vi "Set Exposure Manual.vi"(8 "error in":errorcluster, 11 "DMK33UP2000 in":refnum<class "DMK33UP2000.lvclass">) -> (0 "error out":errorcluster, 2 "Supported?":bool, 3 "DMK33UP2000 out":refnum<class "DMK33UP2000.lvclass">)   [LabVIEW 2018, in "DMK33UP2000.lvlib" / "DMK33UP2000.lvclass"]
uses:
  DMK33UP2000.lvclass
  builds/Camera.lvlibp/Camera.lvclass
  <resource>/objmgr/imaqdx.rc
  C:/Users/Ron.Dexter.LUMINARTECH/Desktop/builds/Camera.lvlibp/Camera.lvclass
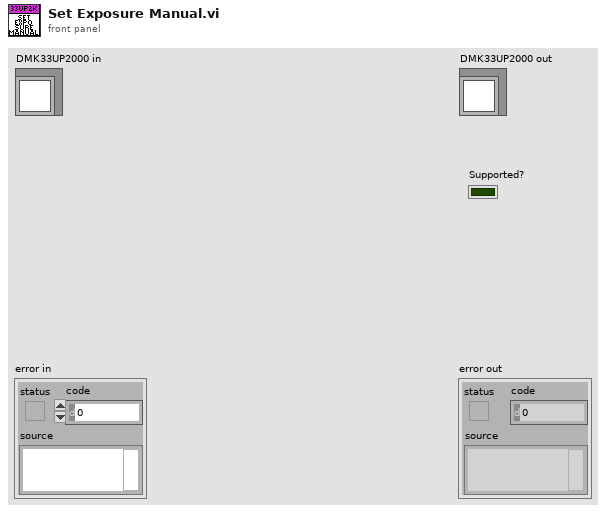
[diagram p1: front panel]
types:
  T1 = typedef "Camera.lvlibp/IMAQdx.ctl" = refnum<k21>
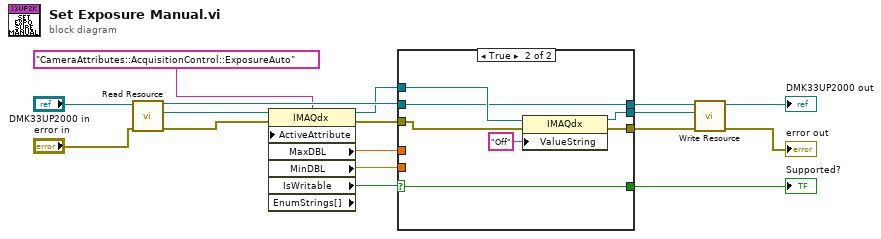
[diagram p0: block diagram]
diagram:
  n1 = call "Read Resource.vi"("error in (no error)"="error in", "Camera in"="DMK33UP2000 in") -> ("error out"=w8:errorcluster, "IMAQdx Session"=w7:T1, "Camera out"=w12:refnum<class "DMK33UP2000.lvclass">)  [unwired: 7 in]
  n2 = property class="IMAQdx" props=["ActiveAttribute", "MaxDBL", "MinDBL", "IsWritable", "EnumStrings[]"](reference=w7, error in=w8, "ActiveAttribute"="CameraAttributes::AcquisitionControl::ExposureAuto") -> (reference out=w10:T1, error out=w14:errorcluster, "MaxDBL"=w16:dbl, "MinDBL"=w17:dbl, "IsWritable"=w9:bool)  [unwired: 1 out]
  n3 = case shown="True" w9 {
    selector: w9 -> [w19 w28]
    tunnel: [w19 w28] -> w1
    tunnel: w10 -> [w20 w27]
    tunnel: [w20 w26] -> w11
    tunnel: w12 -> [w21 w24]
    tunnel: [w21 w24] -> w13
    tunnel: w14 -> [w18 w23]
    tunnel: [w18 w25] -> w15
    tunnel: w16 -> [_ _]
    tunnel: w17 -> [_ _]
    frame False {
    }
    frame True {
      n4 = property class="IMAQdx"(reference=w27, error in=w23, "ValueString"="Off") -> (reference out=w26:T1, error out=w25:errorcluster)
    }
  }
  "Supported?" <- w1
  n5 = call "Write Resource.vi"("error in (no error)"=w15, "IMAQdx Session"=w11, "Camera in"=w13) -> ("error out"=→"error out":errorcluster, "Camera out"=→"DMK33UP2000 out":refnum<class "DMK33UP2000.lvclass">)  [unwired: 7 in]
